vi "Load Instrument.vi"(8 "error in (no error)":errorcluster, 10 "Configuration in":refnum<class "Configuration.lvclass">, 11 "ManualUI in":refnum<class "ManualUI.lvclass">) -> (0 "error out":errorcluster, 1 "Instrument out":refnum<class "Instruments.lvclass">, 2 "Configuration out":refnum<class "Configuration.lvclass">, 3 "ManualUI out":refnum<class "ManualUI.lvclass">)   [LabVIEW 2023, in "ManualUI.lvlib" / "ManualUI.lvclass"]
uses:
  Library/ManualUI.lvclass
  Library/ManualUI.lvclass/ManualUI.ctl
  builds/Framework/Configuration.lvlibp/Library/Configuration.lvclass
  builds/Instruments/Instruments.lvlibp/Library/Instruments.lvclass
  C:/Users/Public/Documents/Development/builds/Framework/Configuration.lvlibp/Library/Configuration.lvclass
  C:/Users/Public/Documents/Development/builds/Framework/Engine.lvlibp/Managed Actor/Library/Managed Actor.lvclass
  C:/Users/Public/Documents/Development/builds/Framework/Engine.lvlibp/Engine/Library/Engine.lvclass
  C:/Users/Public/Documents/Development/builds/Framework/Panel Manager.lvlibp/Library/Panel Actor.lvclass
  C:/Users/Public/Documents/Development/builds/Framework/Monitored Actor.lvlibp/Actor Monitor/Actor Monitor/Actor Monitor.lvclass
  C:/Users/Public/Documents/Development/builds/Framework/Actor Framework.lvlibp/1abvi3w/vi.lib/ActorFramework/Actor/Actor.lvclass
  C:/Users/Public/Documents/Development/builds/Instruments/Instruments.lvlibp/Library/Instruments.lvclass
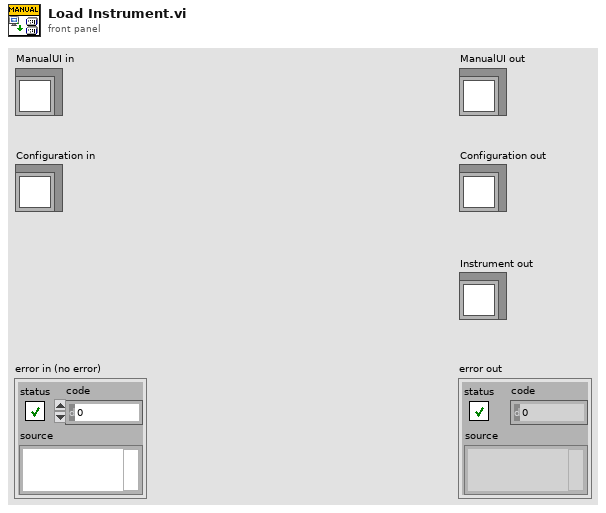
[diagram p1: front panel]
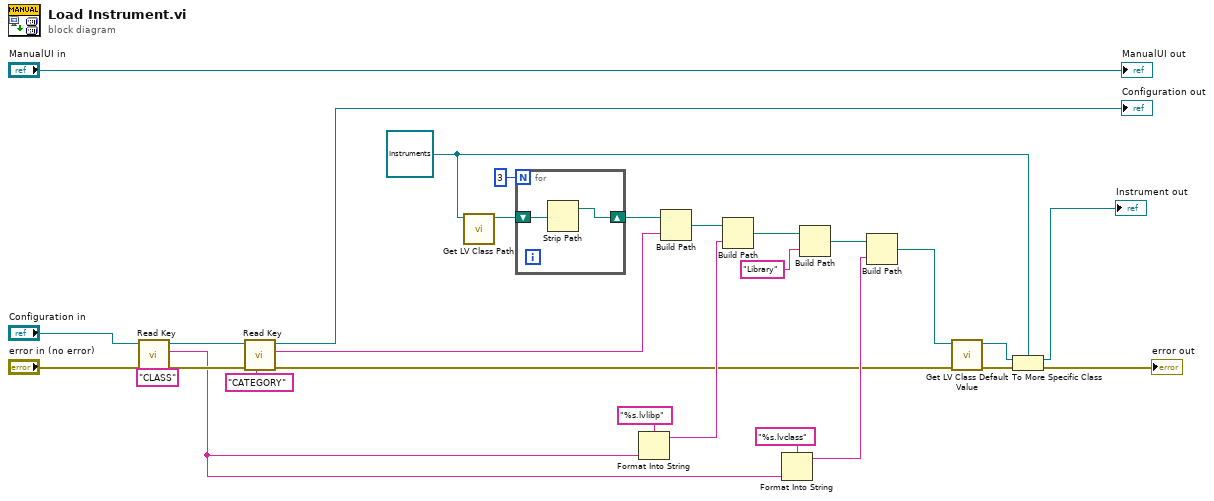
[diagram p0: block diagram]
diagram:
  w4 = refnum<class "Instruments.lvclass"> refnum ("Instrument out")
  n1 = call "Read Key.vi"("Key"="CLASS", "error in (no error)"="error in (no error)", "Configuration in"="Configuration in") -> ("error out"=w22:errorcluster, "Value"=w9:string, "Configuration out"=w20:refnum<class "Configuration.lvclass">)  [unwired: 6 in]
  n2 = call "Read Key.vi"("Key"="CATEGORY", "error in (no error)"=w22, "Configuration in"=w20) -> ("error out"=w2:errorcluster, "Value"=w18:string, "Configuration out"=→"Configuration out":refnum<class "Configuration.lvclass">)  [unwired: 6 in]
  n3 = call <vilib>:"Get LV Class Path.vi"("object"=w4) -> ("class path"=w23:path)  [unwired: 9 in, 1 out]
  n4 = for {
    N: 3 -> [_]
    shift-right: [w29] -> w19
    shift-left: w23 -> [w30]
    n5 = Strip Path(path=w30) -> (stripped path=w29:path)  [unwired: 1 out]
  }
  n6 = Format Into String(format string="%s.lvlibp", w9) -> (resulting string=w14:string)  [unwired: 2 in, 1 out]
  n7 = Build Path(base path=w19, name or relative path=w18) -> (appended path=w15:path)
  n8 = Build Path(base path=w15, name or relative path=w14) -> (appended path=w13:path)
  n9 = Format Into String(format string="%s.lvclass", w9) -> (resulting string=w10:string)  [unwired: 2 in, 1 out]
  n10 = Build Path(base path=w13, name or relative path="Library" ("Key")) -> (appended path=w11:path)
  n11 = Build Path(base path=w11, name or relative path=w10) -> (appended path=w8:path)
  n12 = call <vilib>:"Get LV Class Default Value.vi"("error in (no error)"=w2, "class path"=w8) -> ("error out"=w7:errorcluster, "object"=w6:refnum<class>)  [unwired: 8 in]
  n13 = To More Specific Class(target class=w4, reference=w6, error in=w7) -> (specific class reference=→"Instrument out":refnum<class "Instruments.lvclass">, error out=→"error out":errorcluster)
  "ManualUI out" <- "ManualUI in"
